vi "Define Data Channels.vi"() -> (0 "Tag Producer Channels":string[][](array[string]), 1 "FIFO Producer Channels":string[][](array[string]), 2 "Tag Consumer Channels":string[][](array[string]), 3 "FIFO Consumer Channels":string[][](array[string]))   [LabVIEW 2023, in "BLS Cycler Template.lvlib" / "BLS Cycler Template.lvclass"]
uses:
  BLS Cycler Template.lvclass
  BLS Cycler Template.lvclass/BLS Cycler Template.ctl
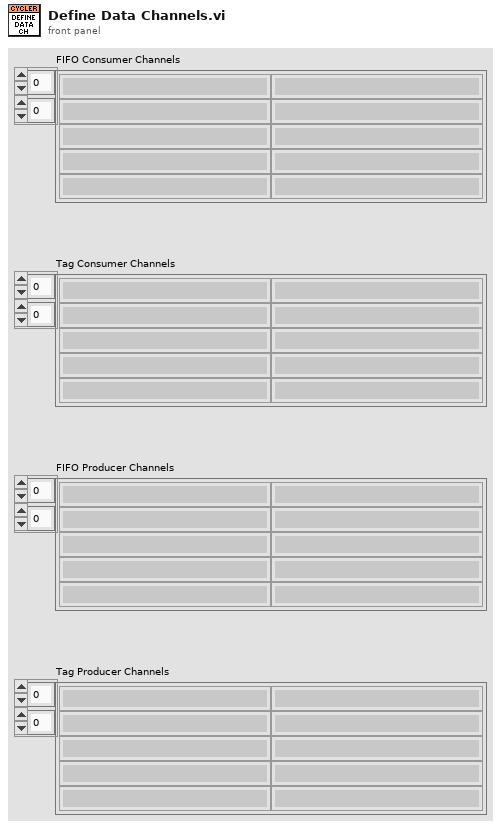
[diagram p1: front panel]
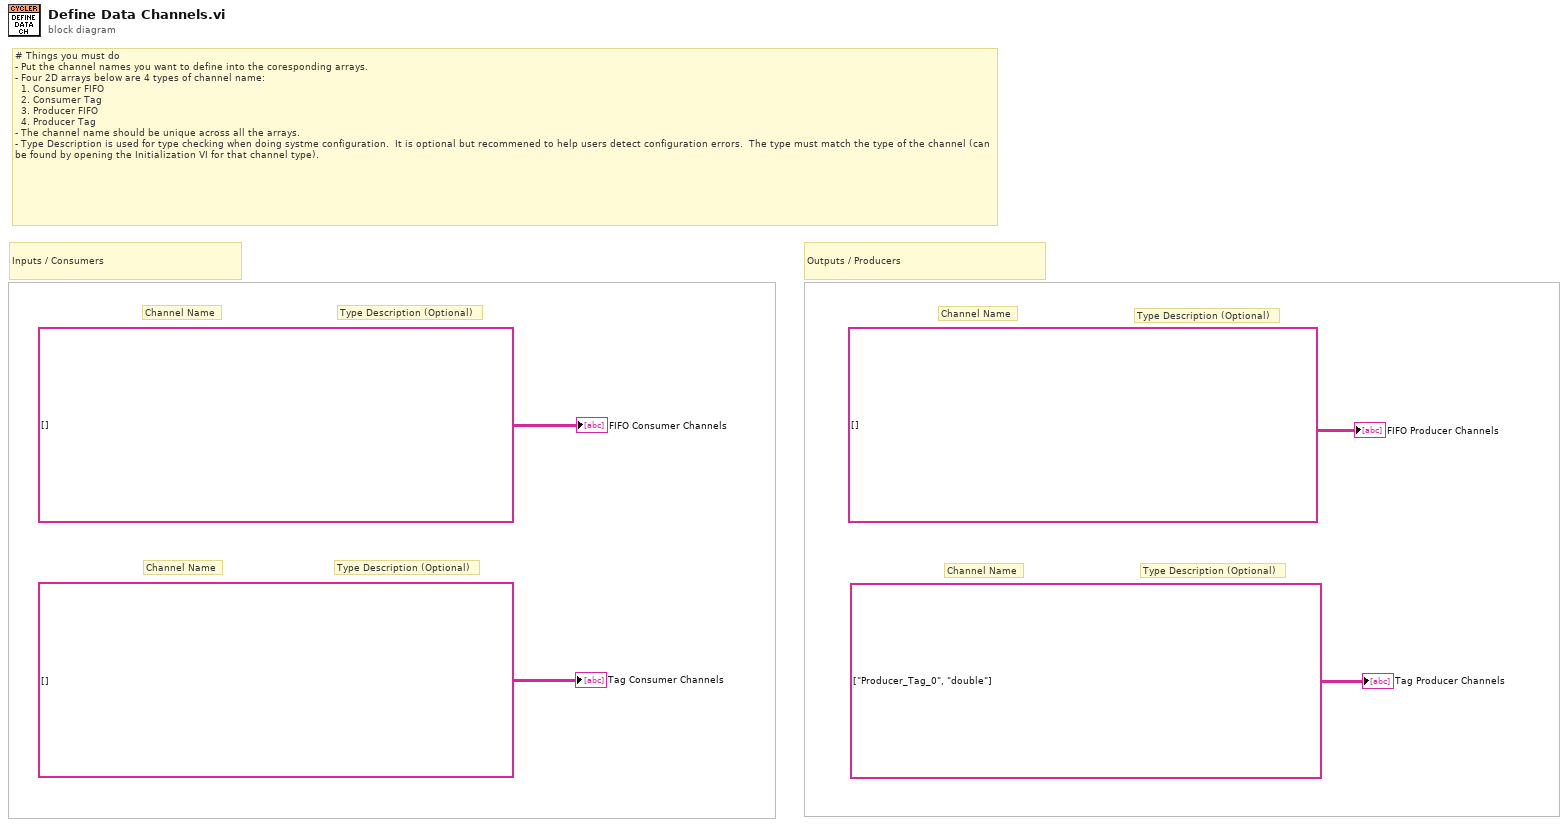
[diagram p0: block diagram]
diagram:
  # "# Things you must do\n- Put the channel names you want to define into the coresponding arrays. \n- Four 2D arrays below are 4 types of channel name:\n  1. Consumer FIFO\n  2. Consumer Tag\n  3. Producer FIFO\n  4. Producer Tag\n- The channel name should be unique across all the arrays.\n- Type Description is used for type checking when doing systme configuration.  It is optional but recommened to help users detect configuration errors.  The type must match the type of the channel (can be found by opening the Initialization VI for that channel type)."
  # "Type Description (Optional)"
  # "Channel Name"
  # "Type Description (Optional)"
  # "Channel Name"
  # "Type Description (Optional)"
  # "Channel Name"
  # "Type Description (Optional)"
  # "Channel Name"
  # "Outputs / Producers"
  # "Inputs / Consumers"
  "FIFO Producer Channels" <- string[][] [] ("Output Channels")
  "FIFO Consumer Channels" <- string[][] [] ("Input Channels")
  "Tag Consumer Channels" <- string[][] [] ("Tag Consumer Channels")
  "Tag Producer Channels" <- string[][] [["Producer_Tag_0", "double"]] ("Tag Producer Channels")
